vi "obj_DataLog Tag Buffers.vi"(0 "method":T2=enum."write", 5 "read index in":i32, 7 "point in":T1 {"value" format="%.3e"; "time" format="%<%H:%M:%S%2u\n%Y/%m/%d>T"}, 9 "tag index":i32=-1, 11 "error in (no error)":errorcluster) -> (4 "available?":bool, 6 "read index out":i32, 8 "point out":T1 {"value" format="%.3e"; "time" format="%<%H:%M:%S%2u\n%Y/%m/%d>T"}, 10 "tag index dup":i32, 15 "error out":errorcluster)   [LabVIEW 2012]
doc: "Provides circular buffers for the tags in the live database. Only the {read} and {read last} methods are intended for public use. All other methods are private.\n\nThe implementation pools the tag buffers so as to provide indexing over tags while avoiding more complicated composite data structures that confuse the LabVIEW compiler sufficiently to not to generate in-place code. By restricting the tag buffers in the pool to have a power of two capacity, modulo the capacity reduces to a simple bitwise \"and\" operation with a mask, and a write or read index overflow (at 2^31) does not invalidate the indexing. To make comparisons of indices overflow insensitve, their difference is compared to zero."
uses:
  typedefs/t_DataLog Tag Buffers Methods.ctl
  typedefs/clusters/t_DataLog Point.ctl
  typedefs/t_DataLog Tag Info List Methods.ctl
  typedefs/t_DataLog Tag Hash Methods.ctl
  typedefs/t_DataLog Tag Expression Evaluator Methods.ctl
  subvis/private/glb_DataLog Runtime Parameterisation.vi
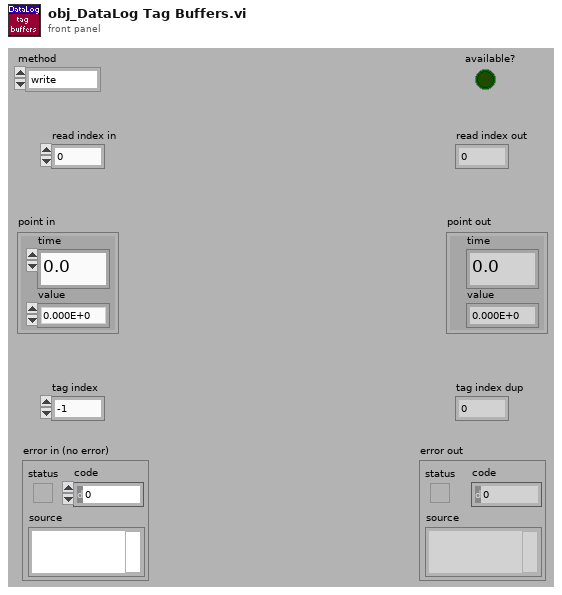
[diagram p1: front panel]
types:
  T1 = typedef "t_DataLog Point.ctl" = cluster{"time":dbl, "value":dbl}
  T2 = typedef "t_DataLog Tag Buffers Methods.ctl" = enum16{"initialize", "inert", "write", "read", "read oldest", "read last", "cleanup"}
  T3 = typedef "t_DataLog Tag Info List Methods.ctl" = enum16{"initialize", "create", "create empty", "rename", "delete", "test tag", "get", "get by name", "get default", "get list", "get path", "get subsets", "set subsets", "set config", "set capacity", "#tags", "go live", "set unlocked", "set mirrored"}
  T4 = typedef "t_DataLog Tag Expression Evaluator Methods.ctl" = enum16{"set", "get", "eval", "assign", "execute", "isvalid", "clear"}
  T5 = typedef "t_DataLog Tag Hash Methods.ctl" = enum16{"initialize", "add tag", "index tag", "lookup", "#tags", "cleanup", "write recovery", "read recovery", "delete recovery"}
  T6 = typedef "t_DataLog Tag Config.ctl" = cluster{"name":string, "unit":string, "temporal":T7, "value":T8, "index":i32, "capacity":i32, "is meta?":bool, "mincapacity":i32, "deadband":dbl, "limit delay":dbl, "format":T9, "precision":u8, "undefine":bool, "update":bool, "update period":u16, "expression":string, "description":string, "logging algorithm":T10, "logging parameters":dbl[]}
  T7 = typedef "t_DataLog Temporal Types.ctl" = enum16{"set&hold", "sample", "event"}
  T8 = typedef "t_DataLog Value Types.ctl" = enum16{"number", "string"}
  T9 = typedef "t_DataLog Numerical Format.ctl" = enum8{"fractional", "exponential", "engineering"}
  T10 = typedef "t_DataLog Logging Algorithms.ctl" = enum16{"nothing", "changes", "everything", "every Nth", "time threshold", "value threshold + prior", "t or v threshold", "t or v threshold + prior"}
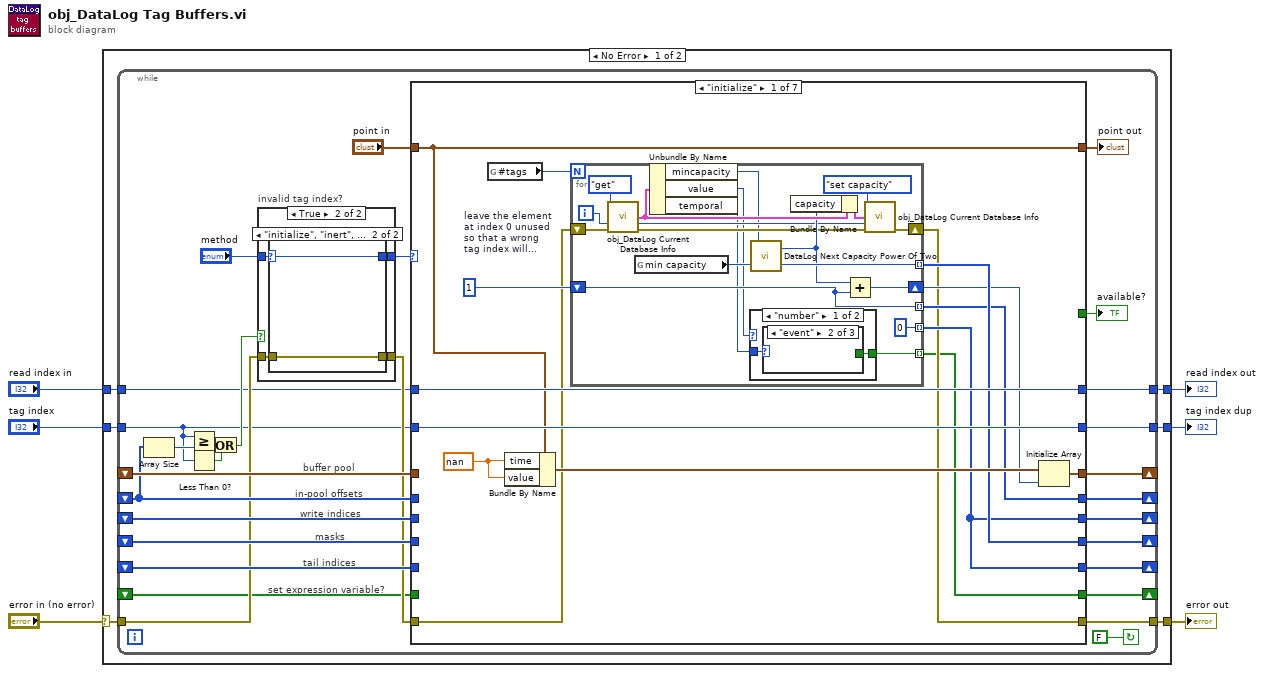
[diagram p0: block diagram]
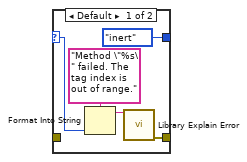
[diagram p3: hidden frame]
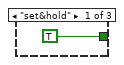
[diagram p4: hidden frame]
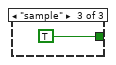
[diagram p5: hidden frame]
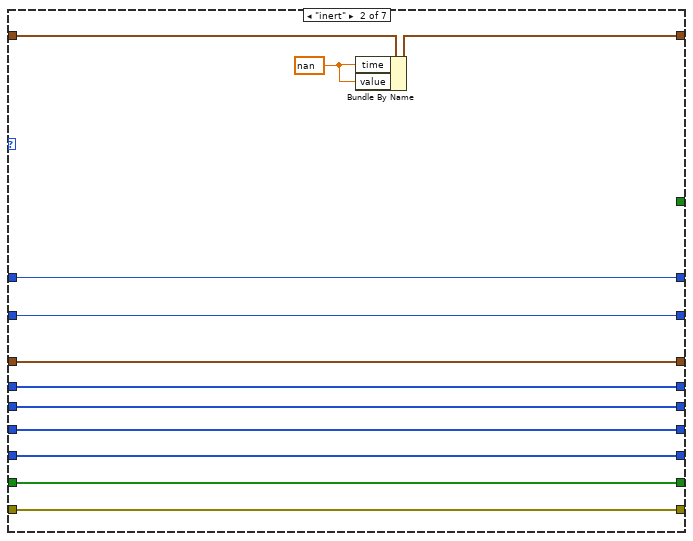
[diagram p7: hidden frame]
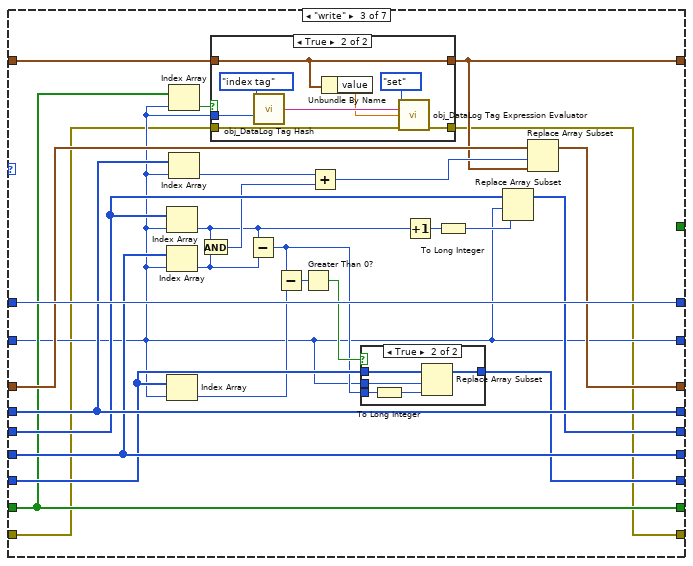
[diagram p8: hidden frame]
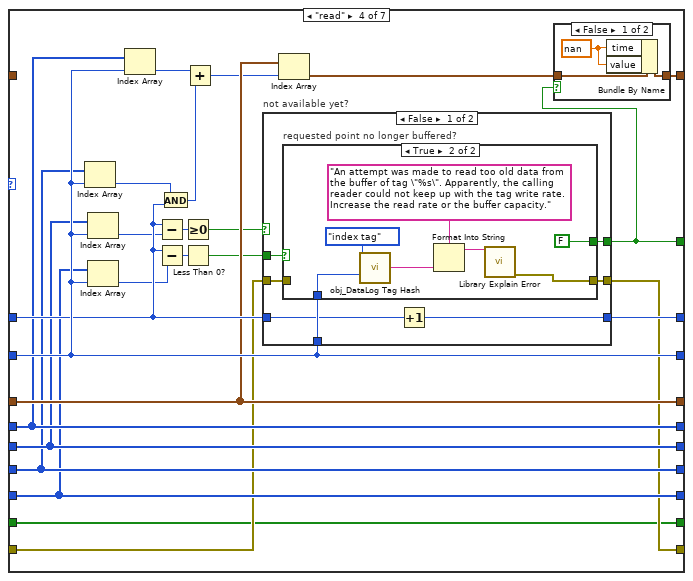
[diagram p11: hidden frame]
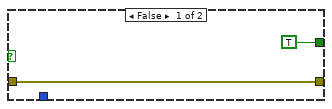
[diagram p13: hidden frame]
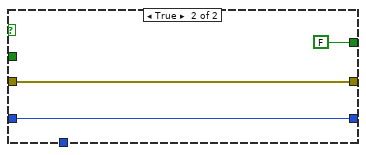
[diagram p14: hidden frame]
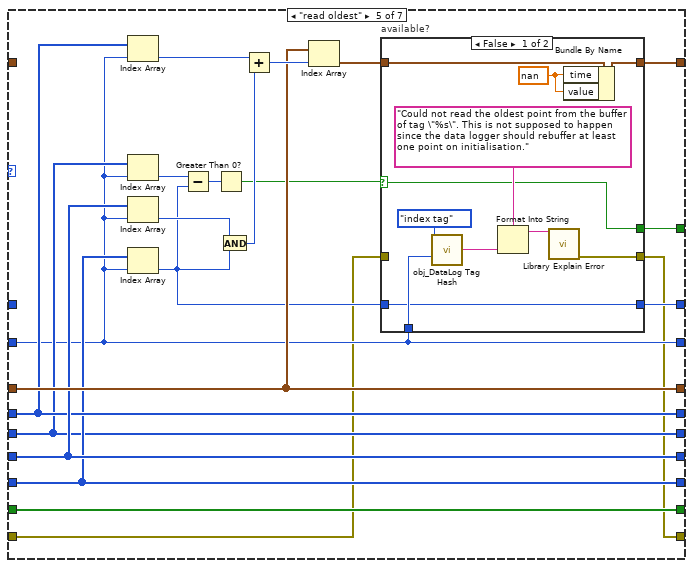
[diagram p15: hidden frame]
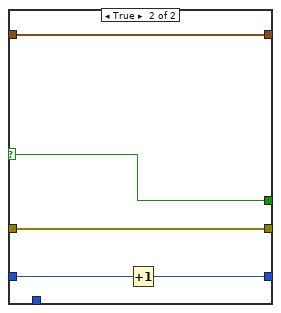
[diagram p16: hidden frame]
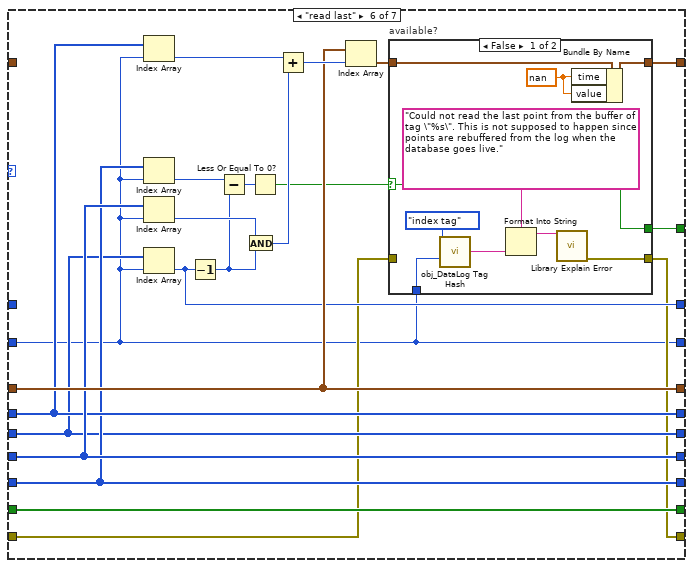
[diagram p17: hidden frame]
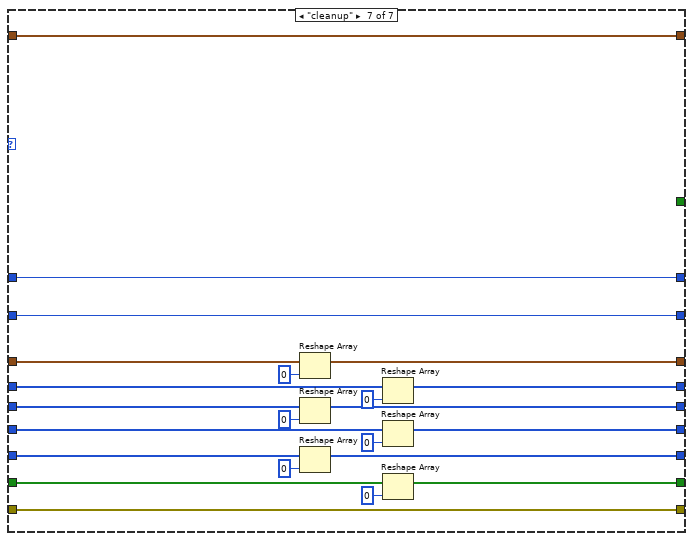
[diagram p19: hidden frame]
diagram:
  n1 = case shown="No Error" "error in (no error)" {
    selector: "error in (no error)" -> [w12 w290]
    tunnel: [w11 w290] -> w5
    tunnel: "read index in" -> [w10 w289]
    tunnel: "tag index" -> [w9 w288]
    tunnel: [w8 w288] -> w2
    tunnel: [w7 w289] -> w1
    frame No Error {
      n2 = while {
        shift-right: [w37] -> _
        shift-left: _ -> [w36]
        shift-right: [w40] -> _
        shift-left: _ -> [w39]
        shift-right: [w38] -> _
        shift-left: _ -> [w26]
        shift-right: [w34] -> _
        shift-left: _ -> [w35]
        tunnel: w12 -> [w23]
        tunnel: [w33] -> w11
        shift-right: [w31] -> _
        shift-left: _ -> [w32]
        tunnel: w10 -> [w18]
        tunnel: w9 -> [w17]
        tunnel: [w16] -> w8
        tunnel: [w15] -> w7
        shift-right: [w13] -> _
        shift-left: _ -> [w14]
        stop <- FALSE continue-if-true
        # "set expression variable?"
        # "tail indices"
        # "masks"
        # "write indices"
        # "in-pool offsets"
        # "buffer pool"
        n3 = Array Size(array=w26) -> (size(s)=w27:i32)
        n4 = Greater Or Equal?(x=w17, y=w27) -> (x >= y?=w25:bool)
        n5 = Less Than 0?(x=w17) -> (x < 0?=w24:bool)
        n6 = Or(x=w25, y=w24) -> (x .or. y?=w20:bool)
        n7 = case "invalid tag index?" shown="True" w20 {
          tunnel: w23 -> [w43 w45]
          tunnel: [w43 w44] -> w22
          tunnel: [w42 w46] -> w21
          tunnel: "method" -> [w42 w47]
          frame False {
          }
          frame True {
            n8 = case shown="\"initialize\", \"inert\", \"cleanup\"" w47 {
              selector: w47 -> [w49 w54]
              tunnel: [t_DataLog_Tag_Buffers_Methods."inert" ("method") w54] -> w46
              tunnel: [w51 w53] -> w44
              tunnel: w45 -> [_ w53]
              frame Default {
                n9 = Format Into String(format string="Method \"%s\" failed. The tag index is out of range.", w49) -> (resulting string=w50:string)  [unwired: 2 in, 1 out]
                n10 = call "Library Explain Error.vi"("explanation prefix (none)"=w50) -> ("explained error"=w51:errorcluster)  [unwired: 14 in]
              }
              frame "initialize", "inert", "cleanup" {
              }
            }
          }
        }
        n11 = case shown="\"initialize\"" w21 {
          tunnel: w18 -> [w67 w97 w131 w169 _ _ w286]
          tunnel: w17 -> [w68 w98 w107 w170 w201 w233 w287]
          tunnel: w39 -> [_ w99 w126 w168 w214 w251 w283]
          tunnel: [w62 w99 w125 w168 w214 w251 w282] -> w40
          tunnel: w26 -> [_ w101 w130 w167 w209 w246 w270]
          tunnel: [w64 w101 w130 w167 w209 w246 w269] -> w38
          tunnel: [w59 w103 w123 w166 w207 w242 w278] -> w37
          tunnel: w36 -> [_ w103 w124 w166 w207 w242 w279]
          tunnel: [w68 w98 w107 w170 w201 w233 w287] -> w16
          tunnel: [w67 w97 w131 w171 w199 w241 w286] -> w15
          tunnel: w35 -> [_ w100 w129 w165 w210 w247 w273]
          tunnel: [w65 w100 w129 w165 w210 w247 w272] -> w34
          tunnel: w22 -> [w58 w104 w106 w161 w198 w235 w285]
          tunnel: [w57 w104 w105 w160 w197 w234 w285] -> w33
          tunnel: w32 -> [_ w102 w120 w164 w208 w243 w276]
          tunnel: [w59 w102 w119 w164 w208 w243 w275] -> w31
          tunnel: "point in" -> [w61 w95 w110 _ _ _ w284]
          tunnel: [w61 w94 w109 w151 w196 w239 w284] -> w29
          tunnel: [_ _ _ w150 w195 w232 _] -> w28
          tunnel: w14 -> [_ w93 w108 w148 w204 w236 w267]
          tunnel: [w56 w93 w108 w148 w204 w236 w266] -> w13
          frame "initialize" {
            w60 = nan ("time")
            w66 = 1  # leave the element at index 0 unused so that a wrong tag index will not clobber any data in the pool
            n12 = global read "glb_DataLog Runtime Parameterisation.vi" "#tags"() -> (w55:i32)
            n13 = Bundle By Name(cluster=w61, "time"=w60, "value"=w60) -> (w69:T1)
            n14 = for {
              N: w55 -> [_]
              shift-right: [w87] -> w63
              shift-left: w66 -> [w86]
              tunnel: [w86] -> w64 mode=indexing
              tunnel: [w81] -> w65 mode=indexing
              tunnel: [0] -> w59 mode=indexing
              shift-right: [w74] -> w57
              shift-left: w58 -> [w76]
              tunnel: [w70] -> w56 mode=indexing
              i -> [w84]
              n15 = call "obj_DataLog Current Database Info.vi"("method"=t_DataLog_Tag_Info_List_Methods."get", "tag index/change#"=w84, "error in (no error)"=w76) -> ("tag config out"=w82:T6, "dup tag index"=w77:i32, "error out"=w75:errorcluster)  [unwired: 6 in, 4 out]
              n16 = global read "glb_DataLog Runtime Parameterisation.vi" "min capacity"() -> (w83:i32)
              n17 = Unbundle By Name(w82) -> ("mincapacity"=w71:i32, "value"=w73:T8, "temporal"=w72:T7)
              n18 = case shown="\"number\"" w73 {
                tunnel: w72 -> [w90 _]
                tunnel: [w89 _] -> w70
                frame "number" {
                  n19 = case shown="\"event\"" w90 {
                    tunnel: [TRUE _ TRUE] -> w89
                    frame "set&hold" {
                    }
                    frame "event" {
                    }
                    frame "sample" {
                    }
                  }
                }
                frame "string" {
                }
              }
              n20 = call "DataLog Next Capacity Power Of Two.vi"("lower limit"=w83, "min capacity"=w71) -> ("mask (2^N-1)"=w81:i32, "actual capacity (2^N)"=w80:i32)
              n21 = Bundle By Name(cluster=w82, "capacity"=w80) -> (w78:T6)
              n22 = Add(x=w80, y=w86) -> (x+y=w87:i32)
              n23 = call "obj_DataLog Current Database Info.vi"("method"=t_DataLog_Tag_Info_List_Methods."set capacity", "tag config in"=w78, "tag index/change#"=w77, "error in (no error)"=w75) -> ("error out"=w74:errorcluster)  [unwired: 5 in, 6 out]
            }
            n24 = Initialize Array(w69, w63) -> (w62:T1[])
          }
          frame "inert" {
            w96 = nan ("time")
            n25 = Bundle By Name(cluster=w95, "time"=w96, "value"=w96) -> (w94:T1)
          }
          frame "write" {
            n26 = Index Array(array=w124, index=w107) -> (element=w117:i32)
            n27 = Index Array(array=w129, index=w107) -> (element=w116:i32)
            n28 = Index Array(array=w120, index=w107) -> (element=w115:i32)
            n29 = Index Array(array=w108, index=w107) -> (element=w111:bool)
            n30 = Index Array(array=w130, index=w107) -> (element=w128:i32)
            n31 = And(x=w117, y=w116) -> (x .and. y?=w122:i32)
            n32 = case shown="True" w111 {
              tunnel: w110 -> [w133 w137]
              tunnel: [w133 w137] -> w109
              tunnel: w107 -> [_ w140]
              tunnel: w106 -> [w132 w135]
              tunnel: [w132 w134] -> w105
              frame False {
              }
              frame True {
                n33 = call "obj_DataLog Tag Hash.vi"("method"=t_DataLog_Tag_Hash_Methods."index tag", "tag index in"=w140) -> ("tag out"=w139:string)  [unwired: 10 in, 3 out]
                n34 = Unbundle By Name(w137) -> ("value"=w136:dbl)
                n35 = call "obj_DataLog Tag Expression Evaluator.vi"("method"=t_DataLog_Tag_Expression_Evaluator_Methods."set", "variable"=w139, "value in"=w136, "error in (no error)"=w135) -> ("error out"=w134:errorcluster)  [unwired: 10 in, 1 out]
              }
            }
            n36 = Subtract(x=w117, y=w116) -> (x-y=w112:i32)
            n37 = Subtract(x=w112, y=w115) -> (x-y=w114:i32)
            n38 = Greater Than 0?(x=w114) -> (x > 0?=w113:bool)
            n39 = Add(x=w128, y=w122) -> (x+y=w127:i32)
            n40 = case shown="True" w113 {
              tunnel: w120 -> [w142 w147]
              tunnel: [w142 w146] -> w119
              tunnel: w112 -> [_ w145]
              tunnel: w107 -> [_ w144]
              frame False {
              }
              frame True {
                n41 = To Long Integer(number=w145) -> (32bit integer=w143:i32)
                n42 = Replace Array Subset(array=w147, new element=w143, index=w144) -> (w146:i32[])
              }
            }
            n43 = Increment(x=w117) -> (x+1=w118:i32)
            n44 = To Long Integer(number=w118) -> (32bit integer=w121:i32)
            n45 = Replace Array Subset(array=w124, new element=w121, index=w107) -> (w123:i32[])
            n46 = Replace Array Subset(array=w126, new element=w109, index=w127) -> (w125:T1[])
          }
          frame "read" {
            n47 = Index Array(array=w165, index=w170) -> (element=w152:i32)
            n48 = Index Array(array=w166, index=w170) -> (element=w158:i32)
            n49 = Index Array(array=w164, index=w170) -> (element=w154:i32)
            n50 = Index Array(array=w167, index=w170) -> (element=w163:i32)
            n51 = Subtract(x=w169, y=w158) -> (x-y=w157:i32)
            n52 = Subtract(x=w169, y=w154) -> (x-y=w159:i32)
            n53 = And(x=w152, y=w169) -> (x .and. y?=w162:i32)
            n54 = Greater Or Equal To 0?(x=w157) -> (x >= 0?=w155:bool)
            n55 = Less Than 0?(x=w159) -> (x < 0?=w156:bool)
            n56 = Add(x=w163, y=w162) -> (x+y=w153:i32)
            n57 = case "not available yet?" shown="False" w155 {
              tunnel: w161 -> [w182 w194]
              tunnel: [w181 w194] -> w160
              tunnel: w156 -> [w180 _]
              tunnel: [w179 FALSE] -> w150
              tunnel: w170 -> [w178 _]
              tunnel: w169 -> [w177 w192]
              tunnel: [w176 w192] -> w171
              frame False {
                n58 = case "requested point no longer buffered?" shown="True" w180 {
                  tunnel: w182 -> [w184 _]
                  tunnel: [w184 w188] -> w181
                  tunnel: [TRUE FALSE] -> w179
                  tunnel: w178 -> [_ w187]
                  frame False {
                  }
                  frame True {
                    n59 = call "obj_DataLog Tag Hash.vi"("method"=t_DataLog_Tag_Hash_Methods."index tag", "tag index in"=w187) -> ("tag out"=w185:string)  [unwired: 10 in, 3 out]
                    n60 = Format Into String(format string="An attempt was made to read too old data from the buffer of tag \"%s\". Apparently, the calling reader could not keep up with the tag write rate. Increase the read rate or the buffer capacity.", w185) -> (resulting string=w190:string)  [unwired: 2 in, 1 out]
                    n61 = call "Library Explain Error.vi"("explanation prefix (none)"=w190) -> ("explained error"=w188:errorcluster)  [unwired: 14 in]
                  }
                }
                n62 = Increment(x=w177) -> (x+1=w176:i32)
              }
              frame True {
              }
            }
            n63 = Index Array(array=w168, index=w153) -> (element=w149:T1)
            n64 = case shown="False" w150 {
              tunnel: w149 -> [w173 w175]
              tunnel: [w172 w175] -> w151
              frame False {
                w174 = nan ("time")
                n65 = Bundle By Name(cluster=w173, "time"=w174, "value"=w174) -> (w172:T1)
              }
              frame True {
              }
            }
          }
          frame "read oldest" {
            n66 = Index Array(array=w209, index=w201) -> (element=w213:i32)
            n67 = Index Array(array=w207, index=w201) -> (element=w205:i32)
            n68 = Index Array(array=w210, index=w201) -> (element=w211:i32)
            n69 = Index Array(array=w208, index=w201) -> (element=w200:i32)
            n70 = Subtract(x=w205, y=w200) -> (x-y=w206:i32)
            n71 = Greater Than 0?(x=w206) -> (x > 0?=w203:bool)
            n72 = And(x=w211, y=w200) -> (x .and. y?=w212:i32)
            n73 = Add(x=w213, y=w212) -> (x+y=w215:i32)
            n74 = Index Array(array=w214, index=w215) -> (element=w202:T1)
            n75 = case "available?" shown="False" w203 {
              selector: w203 -> [w216 w227]
              tunnel: w202 -> [w225 w231]
              tunnel: [w224 w231] -> w196
              tunnel: w198 -> [_ w230]
              tunnel: [w219 w230] -> w197
              tunnel: w201 -> [w218 _]
              tunnel: w200 -> [w217 w229]
              tunnel: [w217 w228] -> w199
              tunnel: [w216 w227] -> w195
              frame False {
                w226 = nan ("time")
                n76 = call "obj_DataLog Tag Hash.vi"("method"=t_DataLog_Tag_Hash_Methods."index tag", "tag index in"=w218) -> ("tag out"=w220:string)  [unwired: 10 in, 3 out]
                n77 = Format Into String(format string="Could not read the oldest point from the buffer of tag \"%s\". This is not supposed to happen since the data logger should rebuffer at least one point on initialisation.", w220) -> (resulting string=w222:string)  [unwired: 2 in, 1 out]
                n78 = call "Library Explain Error.vi"("explanation prefix (none)"=w222) -> ("explained error"=w219:errorcluster)  [unwired: 14 in]
                n79 = Bundle By Name(cluster=w225, "time"=w226, "value"=w226) -> (w224:T1)
              }
              frame True {
                n80 = Increment(x=w229) -> (x+1=w228:i32)
              }
            }
          }
          frame "read last" {
            n81 = Index Array(array=w246, index=w233) -> (element=w250:i32)
            n82 = Index Array(array=w243, index=w233) -> (element=w244:i32)
            n83 = Index Array(array=w247, index=w233) -> (element=w248:i32)
            n84 = Index Array(array=w242, index=w233) -> (element=w241:i32)
            n85 = Decrement(x=w241) -> (x-1=w240:i32)
            n86 = Subtract(x=w244, y=w240) -> (x-y=w245:i32)
            n87 = And(x=w248, y=w240) -> (x .and. y?=w249:i32)
            n88 = Less Or Equal To 0?(x=w245) -> (x <= 0?=w237:bool)
            n89 = Add(x=w250, y=w249) -> (x+y=w252:i32)
            n90 = Index Array(array=w251, index=w252) -> (element=w238:T1)
            n91 = case "available?" shown="False" w237 {
              selector: w237 -> [w253 w263]
              tunnel: w238 -> [w261 w265]
              tunnel: [w260 w265] -> w239
              tunnel: w235 -> [_ w264]
              tunnel: [w255 w264] -> w234
              tunnel: w233 -> [w254 _]
              tunnel: [w253 w263] -> w232
              frame False {
                w262 = nan ("time")
                n92 = call "obj_DataLog Tag Hash.vi"("method"=t_DataLog_Tag_Hash_Methods."index tag", "tag index in"=w254) -> ("tag out"=w256:string)  [unwired: 10 in, 3 out]
                n93 = Format Into String(format string="Could not read the last point from the buffer of tag \"%s\". This is not supposed to happen since points are rebuffered from the log when the database goes live.", w256) -> (resulting string=w258:string)  [unwired: 2 in, 1 out]
                n94 = call "Library Explain Error.vi"("explanation prefix (none)"=w258) -> ("explained error"=w255:errorcluster)  [unwired: 14 in]
                n95 = Bundle By Name(cluster=w261, "time"=w262, "value"=w262) -> (w260:T1)
              }
              frame True {
              }
            }
          }
          frame "cleanup" {
            n96 = Reshape Array(w283, 0 ("dimension size")) -> (w282:T1[])
            n97 = Reshape Array(w279, 0 ("dimension size")) -> (w278:i32[])
            n98 = Reshape Array(w276, 0 ("dimension size")) -> (w275:i32[])
            n99 = Reshape Array(w270, 0 ("dimension size")) -> (w269:i32[])
            n100 = Reshape Array(w273, 0 ("dimension size")) -> (w272:i32[])
            n101 = Reshape Array(w267, 0 ("dimension size")) -> (w266:bool[])
          }
        }
        "point out" <- w29
        "available?" <- w28
      }
    }
    frame Error {
    }
  }
  "error out" <- w5
  "read index out" <- w1
  "tag index dup" <- w2
